vi "lab_2.vi"() -> ()   [LabVIEW 2016]
uses:
  <vilib>/myRIO/Instrument Drivers/Onboard Devices/Accelerometer/typedefs/Accelerometer Reference.ctl
  <vilib>/myRIO/Common/Instrument Driver Framework/Utilities/typedefs/myRIO Generic Hardware Reference.ctl
  <vilib>/myRIO/Common/Instrument Driver Framework/Utilities/typedefs/Hardware Version Enum.ctl
  <vilib>/myRIO/Common/Instrument Driver Framework/Utilities/typedefs/myRIO v1.0 Reference.ctl
  <vilib>/myRIO/Common/Instrument Driver Framework/Utilities/typedefs/Generic FPGA Reference.ctl
  <vilib>/myRIO/Common/Instrument Driver Framework/myRIO v1.0/Accelerometer/typedefs/Accelerometer Channels List.ctl
  <vilib>/myRIO/Common/Instrument Driver Framework/myRIO v1.0/Accelerometer/typedefs/Accelerometer Channels Enum.ctl
  <vilib>/userdefined/High Color/nirio_resource_hc.ctl
  <vilib>/myRIO/Common/Instrument Driver Framework/Utilities/vis/Is FPGA Ref Available.vi
  <vilib>/myRIO/Common/Instrument Driver Framework/myRIO v1.0/Accelerometer/vis/myRIO v1.1 Open Accelerometer.vi
  <vilib>/myRIO/Instrument Drivers/Onboard Devices/Accelerometer/vis/Read.vi
  <vilib>/myRIO/Common/Instrument Driver Framework/Utilities/vis/Validate Channels.vi
  <vilib>/myRIO/Common/Instrument Driver Framework/myRIO v1.0/Accelerometer/vis/myRIO v1.0 Reserve Accelerometer.vi
  <vilib>/myRIO/Common/Instrument Driver Framework/myRIO v1.0/UART/vis/myRIO v1.0 Close UART.vi
  <vilib>/myRIO/Common/Instrument Driver Framework/myRIO v1.0/Resource Manager/vis/myRIO v1.0 Reserve Channel List.vi
  <vilib>/myRIO/Common/Instrument Driver Framework/myRIO v1.0/Accelerometer/vis/myRIO v1.0 Build MUX Configuration Accelerometer.vi
  <vilib>/myRIO/Common/Instrument Driver Framework/myRIO v1.0/Resource Manager/vis/myRIO v1.0 Reserve Channel.vi
  <vilib>/myRIO/Common/Instrument Driver Framework/myRIO v1.0/Resource Manager/vis/myRIO v1.0 Unreserve Channel.vi
  <vilib>/myRIO/Common/Instrument Driver Framework/myRIO v1.0/Resource Manager/vis/myRIO v1.0 Build Mutex Name.vi
  <vilib>/Utility/VariantDataType/GetNumericInfo.vi
  <vilib>/Utility/error.llb/Error Cluster From Error Code.vi
  <vilib>/myRIO/Common/Instrument Driver Framework/myRIO v1.0/myRIO v1.1 Open.vi
  <vilib>/myRIO/Common/Instrument Driver Framework/myRIO v1.0/Accelerometer/vis/myRIO v1.0 Get Scaling Constant Accelerometer.vi
  <vilib>/myRIO/Common/Instrument Driver Framework/Utilities/vis/IO Manager.vi
  <vilib>/myRIO/Common/Instrument Driver Framework/Utilities/vis/Configuration Manager.vi
  <vilib>/myRIO/Common/Instrument Driver Framework/myRIO v1.0/myRIO v1.0 Close.vi
  <vilib>/myRIO/Common/Instrument Driver Framework/myRIO v1.0/Accelerometer/vis/myRIO v1.0 Read Accelerometer.vi
  <vilib>/myRIO/Common/Instrument Driver Framework/Utilities/vis/FPGA Ref Manager.vi
  <vilib>/myRIO/Common/Instrument Driver Framework/myRIO v1.0/myRIO v1.0 Reset FPGA.vi
  <vilib>/myRIO/Common/Instrument Driver Framework/myRIO v1.0/IRQ/vis/myRIO v1.0 IRQ Info FGV.vi
  <vilib>/myRIO/Common/Instrument Driver Framework/myRIO v1.0/IRQ/vis/myRIO v1.0 Timer IRQ Info FGV.vi
  <vilib>/myRIO/Common/Instrument Driver Framework/myRIO v1.0/IRQ/vis/myRIO v1.0 ISR Agent.vi
  <vilib>/myRIO/Express VI/Onboard Devices/Accelerometer/Accelerometer Express VI.xnode
  <vilib>/myRIO/Instrument Drivers/Onboard Devices/Accelerometer/vis/myRIO Accelerometer Open.xnode
  <vilib>/myRIO/Instrument Drivers/Onboard Devices/Accelerometer/Accelerometer.lvlib
  <vilib>/myRIO/Instrument Drivers/Utilities/Utilities.lvlib
panel:
  out "Data Collection":dbl[][](array[numeric])
  in  "Smoothing Factor":dbl(slide) min=0.0 max=1.0 step=0.05 scale=0.0..1.0
  in  "ON/OFF":bool
  out "MyRIO Angular Position":cluster{dbl, dbl}(graph)
  out "error out":errorcluster
  in  "Main Loop STOP":bool
  out "MyRIO Accelerometer":T1(graph)
  # "Lab 2: Example Submission"
  # "Project features:\n- 3-axis accelerometer instantiation\n- computation of roll and pitch\n- real-time plotting\n- optional low-pass filter with adjustable parameter\n- real-time data collection"
  # "Author: Adam Cavatassi, McGill University, 2018"
  # "Low-Pass Filter"
  # "G_z"
  # "G_y"
  # "G_x"
  # "roll"
  # "pitch"
  # "# Samples"
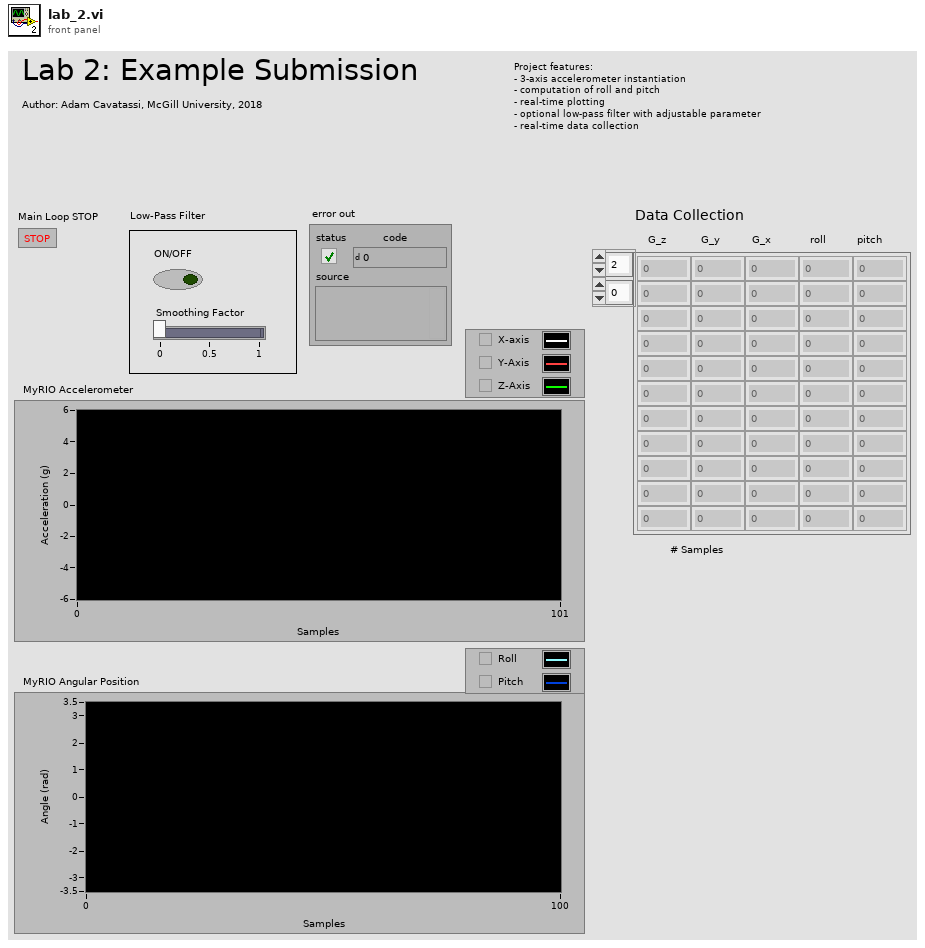
[diagram p1: front panel]
types:
  T1 = cluster{"X-Axis":dbl, "Y-Axis":dbl, "Z-Axis":dbl}
  T2 = typedef "Accelerometer.lvlib/Accelerometer Reference.ctl" = cluster{"myRIO Reference":T3, "Accelerometer Channels List":T7, "LSB Weight":dbl}
  T3 = typedef "myRIO Generic Hardware Reference.ctl" = cluster{"myRIO Model":T4, "myRIO Hardware Reference":T5}
  T4 = typedef "Hardware Version Enum.ctl" = enum16{"Unknown", "myRIO-1900", "myRIO-1950", "roboRIO", "NI ELVIS RIO CM"}
  T5 = typedef "myRIO v1.0 Reference.ctl" = cluster{"Generic FPGA Reference":T6, "Allow multiple opens":bool}
  T6 = typedef "Generic FPGA Reference.ctl" = refnum<k20>
  T7 = typedef "Accelerometer Channels List.ctl" = T8[]
  T8 = typedef "Accelerometer Channels Enum.ctl" = enum16{"Not Connected", "X-Axis", "Y-Axis", "Z-Axis"}
  T9 = typedef "nirio_resource_hc.ctl" = tag
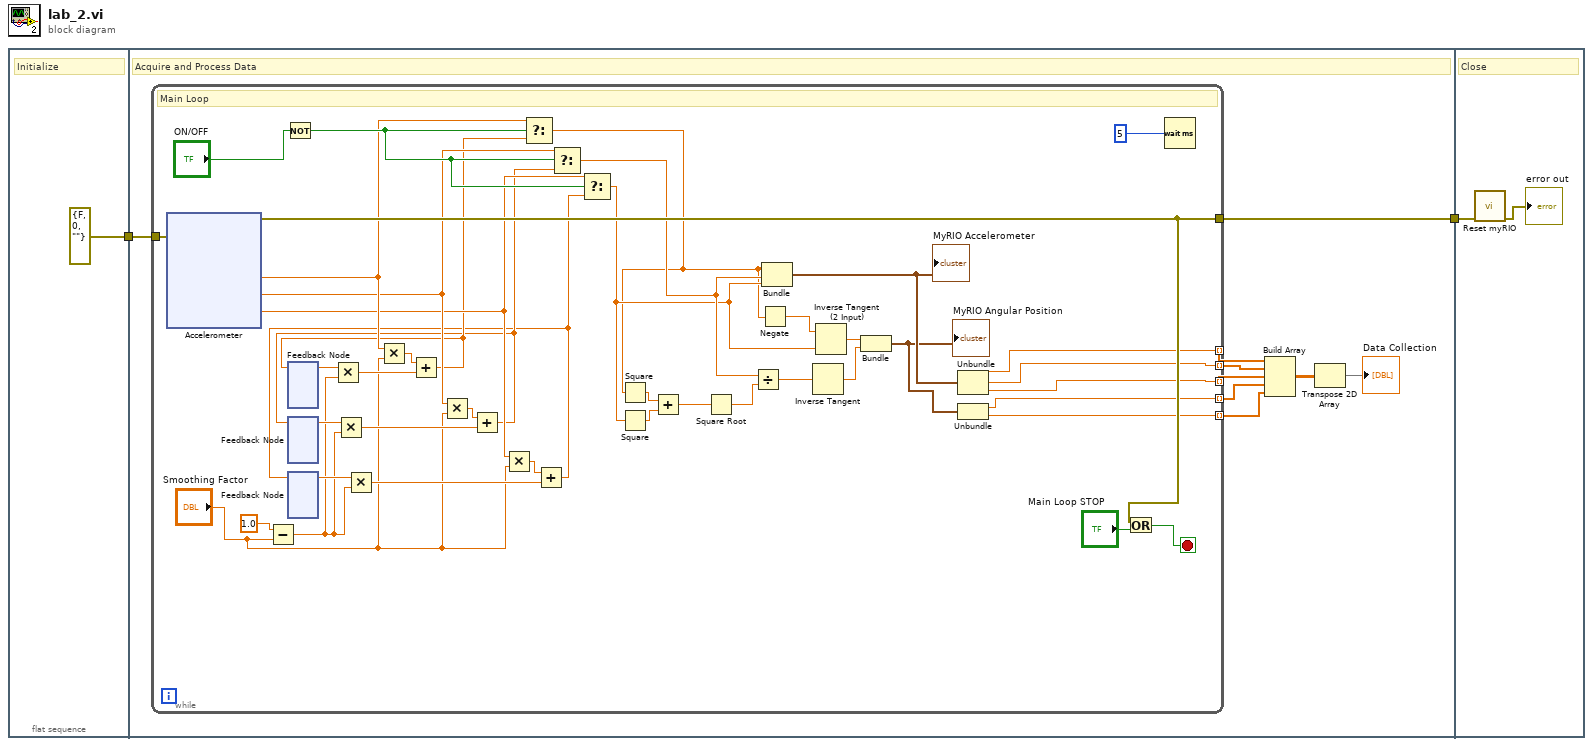
[diagram p0: block diagram]
diagram:
  n1 = flat-sequence {
    tunnel: [errorcluster {"status"=FALSE, "code"=0, "source"=""} ("error in (no error)")] -> w2
    tunnel: w2 -> [w12]
    tunnel: [w11] -> w1
    tunnel: w1 -> [w96]
    frame #0 {
      # "Initialize"
    }
    frame #1 {
      # "Acquire and Process Data"
      n2 = while {
        tunnel: w12 -> [w54]
        tunnel: [w51] -> w11
        tunnel: [w18] -> w10 mode=indexing
        tunnel: [w17] -> w9 mode=indexing
        tunnel: [w16] -> w8 mode=indexing
        tunnel: [w15] -> w7 mode=indexing
        tunnel: [w14] -> w6 mode=indexing
        stop <- w53 stop-if-true
        # "Main Loop"
        n3 = xnode "Accelerometer"("error in (no error)"=w54) -> ("X-Axis"=w30:dbl, "Y-Axis"=w29:dbl, "Z-Axis"=w26:dbl, "error out"=w51:errorcluster)
        n4 = Subtract(x=1.0, y="Smoothing Factor") -> (x-y=w31:dbl)
        n5 = Not(x="ON/OFF") -> (.not. x?=w35:bool)
        n6 = feedback #1() -> (w42:dbl)  [unwired: 1 in]
        n7 = feedback #2() -> (w41:dbl)  [unwired: 1 in]
        n8 = feedback #3() -> (w40:dbl)  [unwired: 1 in]
        n9 = Multiply(x=w42, y=w31) -> (x*y=w34:dbl)
        n10 = Multiply(x=w41, y=w31) -> (x*y=w33:dbl)
        n11 = Multiply(x=w40, y=w31) -> (x*y=w32:dbl)
        n12 = Multiply(x=w30, y="Smoothing Factor") -> (x*y=w27:dbl)
        n13 = Add(x=w27, y=w34) -> (x+y=w24:dbl)
        n14 = feedback-in #1(w24) -> ()
        n15 = Multiply(x=w29, y="Smoothing Factor") -> (x*y=w28:dbl)
        n16 = Add(x=w28, y=w33) -> (x+y=w23:dbl)
        n17 = feedback-in #2(w23) -> ()
        n18 = Multiply(x=w26, y="Smoothing Factor") -> (x*y=w25:dbl)
        n19 = Select(t=w30, s=w35, f=w24) -> (s? t:f=w13:dbl)
        n20 = Add(x=w25, y=w32) -> (x+y=w22:dbl)
        n21 = feedback-in #3(w22) -> ()
        n22 = Select(t=w29, s=w35, f=w23) -> (s? t:f=w38:dbl)
        n23 = Select(t=w26, s=w35, f=w22) -> (s? t:f=w37:dbl)
        n24 = Square(x=w13) -> (x^2=w45:dbl)
        n25 = Square(x=w37) -> (x^2=w50:dbl)
        n26 = Add(x=w45, y=w50) -> (x+y=w49:dbl)
        n27 = Square Root(x=w49) -> (sqrt(x)=w48:dbl)
        n28 = Divide(x=w38, y=w48) -> (x/y=w47:dbl)
        n29 = Negate(x=w13) -> (-x=w44:dbl)
        n30 = Bundle("X-Axis"=w13, "Y-Axis"=w38, "Z-Axis"=w37) -> (w20:T1)  [unwired: 1 in]
        "MyRIO Accelerometer" <- w20
        n31 = Inverse Tangent(1:w47) -> (0:w46:dbl)
        n32 = Inverse Tangent (2 Input)(1:w37, 2:w44) -> (0:w43:dbl)
        n33 = Bundle(w43, w46) -> (w19:cluster{dbl, dbl})  [unwired: 1 in]
        "MyRIO Angular Position" <- w19
        n34 = Unbundle(w20) -> ("X-Axis"=w18:dbl, "Y-Axis"=w17:dbl, "Z-Axis"=w16:dbl)
        n35 = Unbundle(w19) -> (w15:dbl, w14:dbl)
        n36 = Or(x=w51, y="Main Loop STOP") -> (x .or. y?=w53:bool)
        n37 = Wait (ms)(milliseconds to wait=5) -> ()  [unwired: 1 out]
      }
      n38 = Build Array(w10, w9, w8, w7, w6) -> (w5:dbl[][])
      n39 = Transpose 2D Array(2D array=w5) -> (transposed array=→"Data Collection":dbl[][])
    }
    frame #2 {
      # "Close"
      n40 = call <vilib>:"Reset myRIO.vi"("error in (no error)"=w96) -> ("error out"=→"error out":errorcluster)  [unwired: 10 in]
    }
  }
